vi "GroupUI.vi"() -> ()   [LabVIEW 2013, in "device.lvclass"]
uses:
  device.lvclass
  <vilib>/NI/Configuration Framework/Node/NodeRef.ctl
  <vilib>/NI/Configuration Framework/Node/NISE_CEF_Node.lvclass
  <vilib>/NI/AMC/Message Queue.ctl
  <vilib>/NI/AMC/Message.ctl
  <vilib>/NI/Tools/Keyed Array/KeyedArray.ctl
  <vilib>/NI/Configuration Framework/Node/UserEventRef.ctl
  <vilib>/NI/Configuration Framework/Controls/EventCluster.ctl
  database file/signal configuration.ctl
  J1939 Library/Configuration/TypeDefs/J1939 db frame direction.ctl
  device.lvclass/device.ctl
  device registry command.ctl
  <vilib>/NI/AMC/Create Single Message.vi
  <vilib>/NI/AMC/Update Message Routing Info.vi
  database file/J1939FullDB.vi
  <vilib>/NI/AMC/Send Message.vi
  <vilib>/NI/AMC/AMC.lvlib
  database file/database file.lvclass
  <vilib>/NI/Tools/Keyed Array/Tools_KeyedArray.lvlib
  <vilib>/NI/Configuration Framework/NISE_CEF_TreeControl.lvlib
  J1939 Library/J1939.lvlib
panel:
  in  "Direction":T1
  in  "Priority":u8
  in  "Transmit Time":dbl
  in  "Output Timing Type":u32(ring) items=["Cyclic Data", "Event Data"]
  out "information":string
  in  "Signals":T2[](array[typedef])
  in  "remove":bool
  in  "add":bool
  in  "Configured Frames (PGN)":i32(listbox)
  in  "Available Frames (PGN)":i32(listbox)
  in  "Source Address":u8
  in  "user event":T3
  in  "main queue":T4
  in  "node ref":T5
  # "Frame Settings"
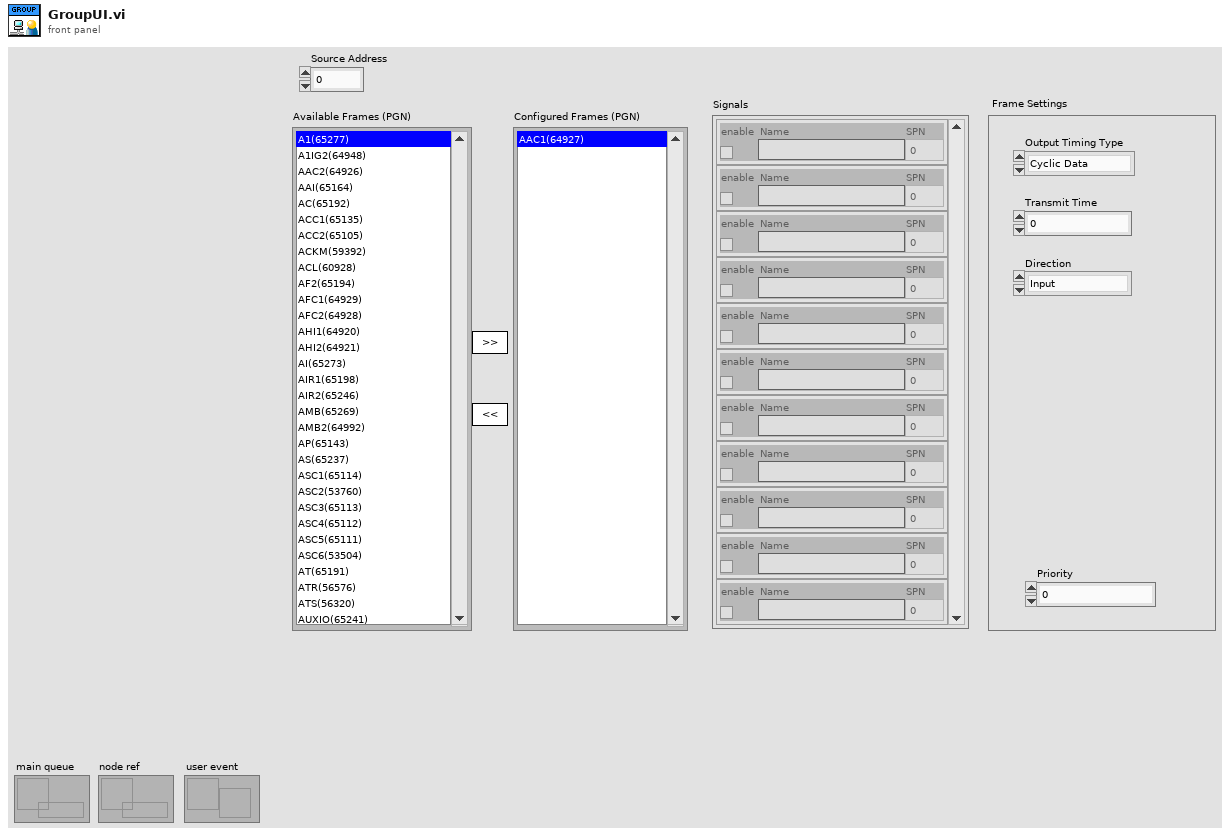
[diagram p1: front panel]
types:
  T1 = typedef "J1939.lvlib/J1939 db frame direction.ctl" = enum16{"Input", "Output", "Input+Output"}
  T2 = typedef "device.lvclass/signal configuration.ctl" = cluster{"enable":bool, "Name":string, "SPN":u32}
  T3 = typedef "NISE_CEF_Node.lvclass/UserEventRef.ctl" = refnum<user-event>
  T4 = typedef "AMC.lvlib/Message Queue.ctl" = refnum<queue>
  T5 = typedef "NISE_CEF_Node.lvclass/NodeRef.ctl" = refnum<data-value>
  T6 = typedef "J1939.lvlib/J1939 db.ctl" = cluster{"BaudRate":u32, "CAN.IoMode":u32, "J1939 Network Address":u8, "Name":u64, "frames":T7[]}
  T7 = typedef "J1939.lvlib/J1939 db frame.ctl" = cluster{"name":string, "Priority":u8, "PGN":u32, "Reserved Bit":u8, "Data page":u8, "PDU Format":u8, "PDU Specific":u8, "Source Address":u8, "PayldLen":u32, "signals":T8[], "Comment":string, "can timing type":u32, "transmit time":dbl, "direction":u16}
  T8 = typedef "J1939.lvlib/J1939 db signal.ctl" = cluster{"NameShort":string, "SPN":i32, "StartBit":u32, "NumBits":u32, "DataType":u32, "ByteOrdr":u32, "ScaleFac":dbl, "ScaleOff":dbl, "Max":dbl, "Min":dbl, "Default":dbl, "Unit":string, "Comment":string}
  T9 = typedef "device.lvclass/device registry command.ctl" = enum16{"add device", "remove device", "get next available"}
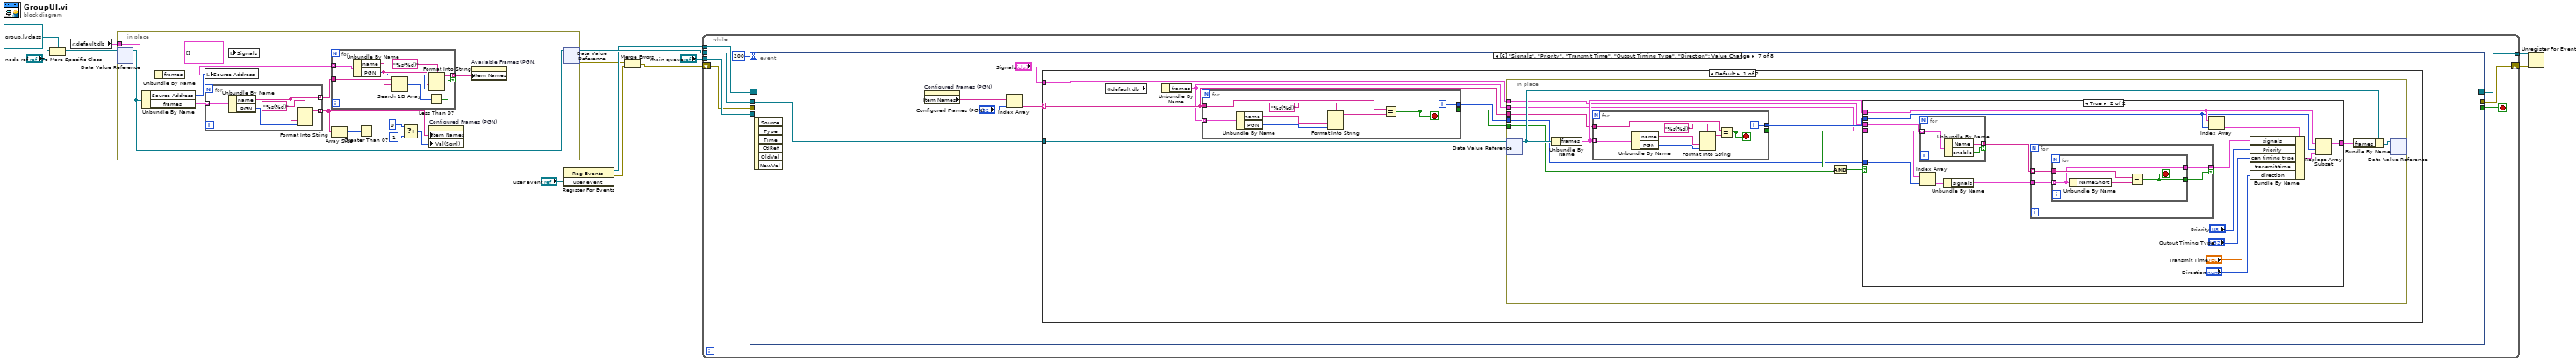
[diagram p0: block diagram]
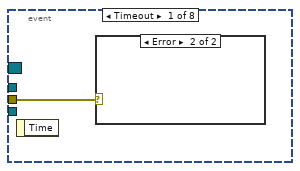
[diagram p2: hidden frame]
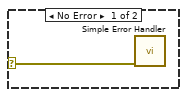
[diagram p3: hidden frame]
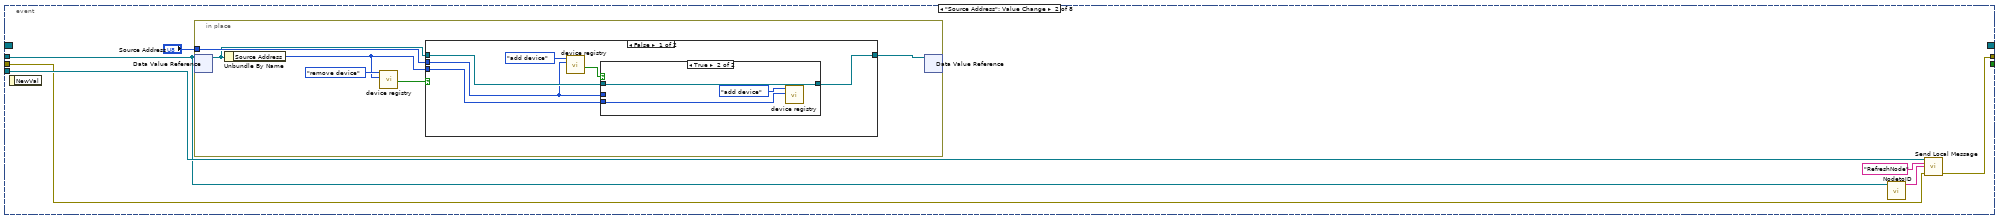
[diagram p4: hidden frame]
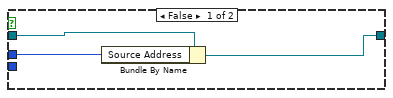
[diagram p5: hidden frame]
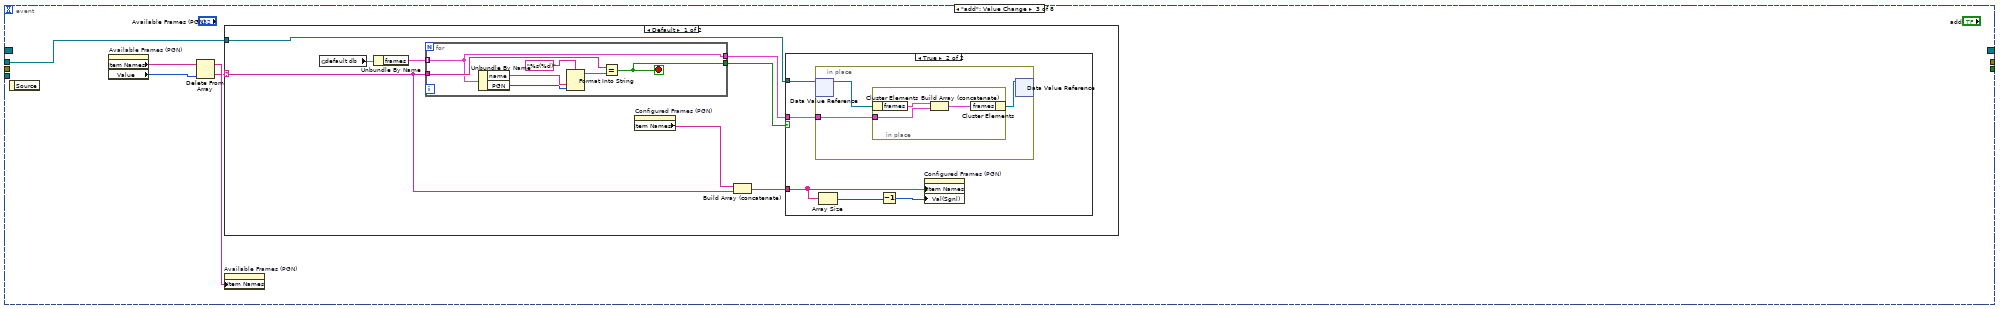
[diagram p7: hidden frame]
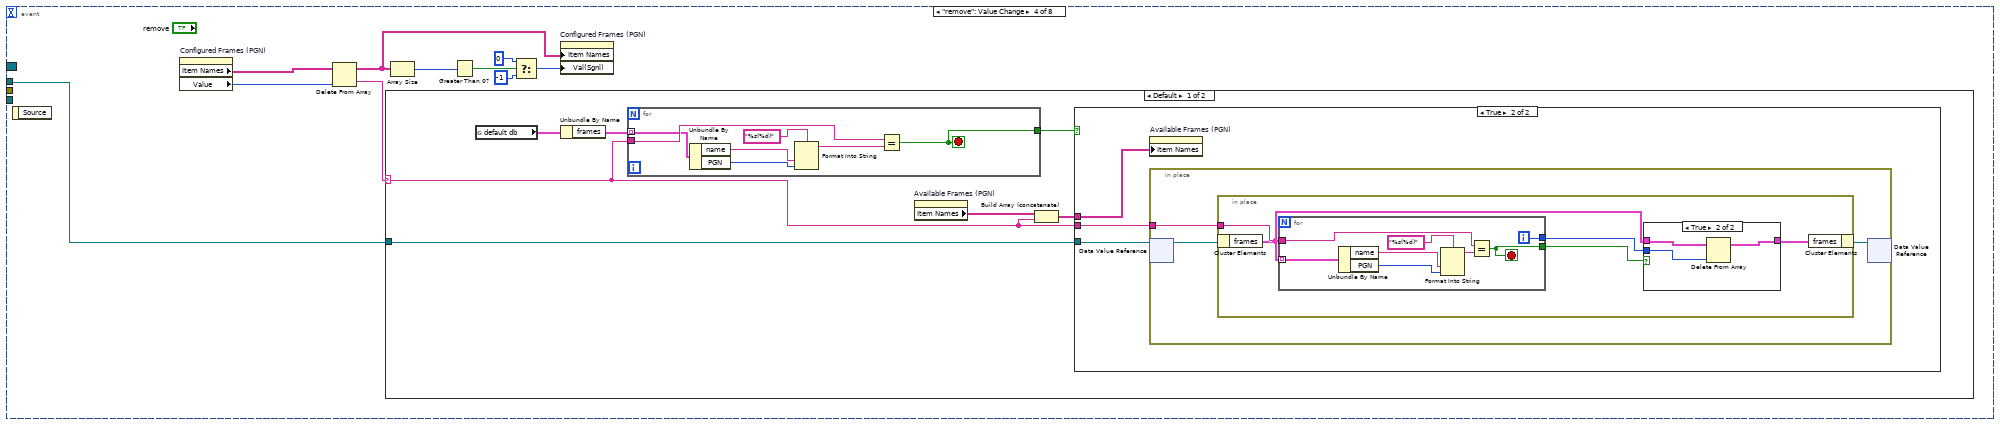
[diagram p10: hidden frame]
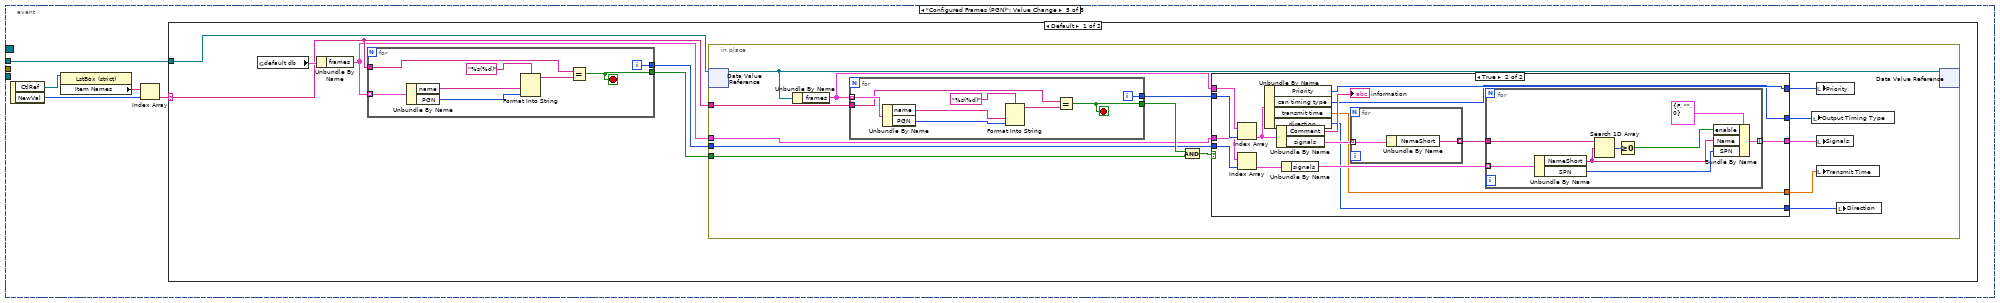
[diagram p14: hidden frame]
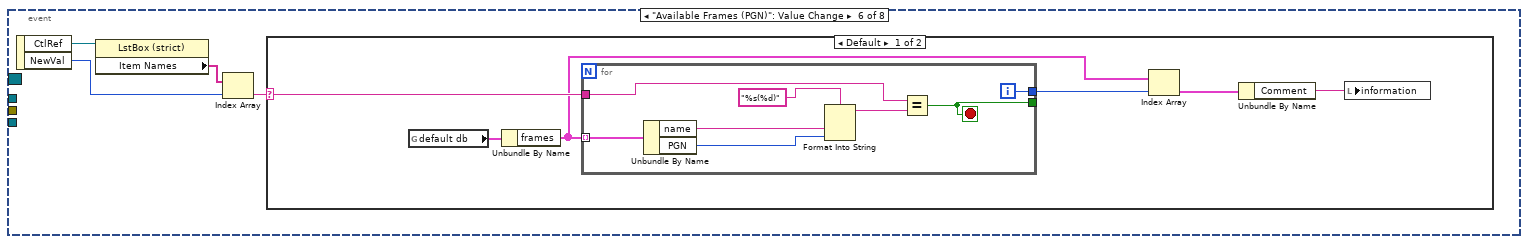
[diagram p17: hidden frame]
diagram:
  n1 = To More Specific Class(target class=refnum<data-value> refnum ("data value reference"), reference="node ref") -> (specific class reference=w6:refnum<data-value>)  [unwired: 1 in, 1 out]
  n2 = global read "J1939FullDB.vi" "default db"() -> (w1:T6)
  n3 = in-place {
    in-place-border: w1 -> [w18]
    n4 = in-place-dvr #1(w6) -> (w27:refnum<class "device.lvclass">)  [unwired: 1 out]
    n5 = Unbundle By Name(w27) -> ("Source Address"=w26:u8, "frames"=w25:T7[])
    n6 = Unbundle By Name(w18) -> ("frames"=w17:T7[])
    n7 = local write "Source Address"(w26) -> ()
    n8 = for {
      tunnel: w25 -> [w40] mode=indexing
      tunnel: [w37] -> w24 mode=indexing
      tunnel: [w36] -> w16 mode=indexing
      n9 = Unbundle By Name(w40) -> ("name"=w36:string, "PGN"=w39:u32)
      n10 = Format Into String(format string="%s(%d)", w36, w39) -> (resulting string=w37:string)  [unwired: 2 in, 1 out]
    }
    n11 = local write "Signals"(T2[] [] ("Signals")) -> ()
    n12 = for {
      tunnel: w17 -> [w35] mode=indexing
      tunnel: w16 -> [w34]
      tunnel: [w30] -> w15 mode=indexing if=w28
      n13 = Unbundle By Name(w35) -> ("name"=w32:string, "PGN"=w31:u32)
      n14 = Search 1D Array(1D array=w34, element=w32) -> (index of element=w29:i32)  [unwired: 1 in]
      n15 = Less Than 0?(x=w29) -> (x < 0?=w28:bool)
      n16 = Format Into String(format string="%s(%d)", w32, w31) -> (resulting string=w30:string)  [unwired: 2 in, 1 out]
    }
    n17 = Array Size(array=w24) -> (size(s)=w23:i32)
    n18 = Greater Than 0?(x=w23) -> (x > 0?=w22:bool)
    n19 = Select(t=0 ("Value (Signaling)"), s=w22, f=-1 ("Value (Signaling)")) -> (s? t:f=w20:i32)
    n20 = property on="Configured Frames (PGN)" class="LstBox (strict)"("Item Names"=w24, "Val(Sgnl)"=w20) -> ()  [unwired: 2 in, 2 out]
    n21 = property on="Available Frames (PGN)" class="LstBox (strict)"("Item Names"=w15) -> ()  [unwired: 2 in, 2 out]
    n22 = in-place-dvr #1(w27) -> (w13:refnum<data-value>, w3:errorcluster)
  }
  n23 = register-events("user event") -> (reference out=w10:refnum<event-registration>, error out=w4:errorcluster)  [unwired: 2 in]
  n24 = Merge Errors(w3, w4) -> (w2:errorcluster)
  n25 = while {
    tunnel: w13 -> [w48]
    tunnel: "main queue" -> [w47]
    tunnel: w10 -> [w45]
    tunnel: [w44] -> w9
    shift-right: [w42] -> w8
    shift-left: w2 -> [w41]
    stop <- w43 stop-if-true
    n26 = event shown="[6] \"Signals\", \"Priority\", \"Transmit Time\", \"Output Timing Type\", \"Direction\": Value Change" {
      selector: w45 -> [_ _ _ _ _ _ _ _]
      dyn-events: [_ _ _ _ _ _ _ _] -> w44
      timeout: 200 -> [_ _ _ _ _ _ _ _]
      tunnel: w48 -> [_ w55 w77 w114 w155 _ w239 _]
      tunnel: w47 -> [_ w56 _ _ _ _ _ _]
      tunnel: [_ _ _ _ _ _ _ TRUE] -> w43
      tunnel: [_ w53 _ _ _ _ _ _] -> w42
      tunnel: w41 -> [w49 w52 _ _ _ _ _ _]
      event Timeout {
        n27 = event-data() -> ()  [unwired: 1 in, 1 out]
        n28 = case shown="Error" w49 {
          selector: w49 -> [w50 _]
          frame No Error {
            n29 = call <vilib>:"Simple Error Handler.vi"("error in (no error)"=w50) -> ()  [unwired: 4 in, 5 out]
          }
          frame Error {
          }
        }
      }
      event "Source Address": Value Change {
        n30 = event-data() -> ()  [unwired: 1 in, 1 out]
        n31 = in-place {
          in-place-border: "Source Address" -> [w62]
          n32 = in-place-dvr #2(w55) -> (w61:refnum<class "device.lvclass">)  [unwired: 1 out]
          n33 = Unbundle By Name(w61) -> ("Source Address"=w58:u8)
          n34 = call "device registry.vi"("device"=w58, "command"=device_registry_command."remove device") -> ("Error?"=w59:bool)  [unwired: 8 in, 1 out]
          n35 = case shown="False" w59 {
            tunnel: [w69 w76] -> w63
            tunnel: w62 -> [w65 _]
            tunnel: w61 -> [w68 w76]
            tunnel: w58 -> [w64 _]
            frame False {
              n36 = call "device registry.vi"("device"=w65, "command"=device_registry_command."add device") -> ("Error?"=w66:bool)  [unwired: 8 in, 1 out]
              n37 = case shown="True" w66 {
                tunnel: [w72 w75] -> w69
                tunnel: w68 -> [w71 w75]
                tunnel: w65 -> [w70 _]
                tunnel: w64 -> [_ w73]
                frame False {
                  n38 = Bundle By Name(cluster=w71, "Source Address"=w70) -> (w72:refnum<class "device.lvclass">)
                }
                frame True {
                  n39 = call "device registry.vi"("device"=w73, "command"=device_registry_command."add device") -> ()  [unwired: 8 in, 2 out]
                }
              }
            }
            frame True {
            }
          }
          n40 = in-place-dvr #2(w63) -> ()  [unwired: 2 out]
        }
        n41 = call <vilib>:"NodetoID.vi"("node ref"=w55) -> ("ID"=w54:string)  [unwired: 9 in, 1 out]
        n42 = call <vilib>:"Send Local Message.vi"("message queue in"=w56, "message name"="RefreshNode" ("Message Name"), "message value"=w54, "error in"=w52) -> ("error out"=w53:errorcluster)  [unwired: 9 in, 2 out]
      }
      event "add": Value Change {
        n43 = event-data() -> ()  [unwired: 1 in, 1 out]
        n44 = property on="Available Frames (PGN)" class="LstBox (strict)"() -> ("Item Names"=w81:string[], "Value"=w80:i32)  [unwired: 2 in, 2 out]
        n45 = Delete From Array(array=w81, index=w80) -> (deleted portion=w78:string, array with subset deleted=w79:string[])  [unwired: 1 in]
        n46 = case shown="Default" w78 {
          selector: w78 -> [w86 _]
          tunnel: w77 -> [w83 _]
          frame Default {
            n47 = global read "J1939FullDB.vi" "default db"() -> (w88:T6)
            n48 = Unbundle By Name(w88) -> ("frames"=w87:T7[])
            n49 = for {
              tunnel: w87 -> [w101] mode=indexing
              tunnel: w86 -> [w103]
              tunnel: [w102] -> w85
              tunnel: [w101] -> w82
              stop <- w102 stop-if-true
              n50 = Unbundle By Name(w101) -> ("name"=w106:string, "PGN"=w105:u32)
              n51 = Format Into String(format string="%s(%d)", w106, w105) -> (resulting string=w104:string)  [unwired: 2 in, 1 out]
              n52 = Equal?(x=w103, y=w104) -> (x = y?=w102:bool)
            }
            n53 = property on="Configured Frames (PGN)" class="LstBox (strict)"() -> ("Item Names"=w89:string[])  [unwired: 2 in, 2 out]
            n54 = Build Array (concatenate)(w89, w86) -> (w84:string[])
            n55 = case shown="True" w85 {
              tunnel: w84 -> [_ w92]
              tunnel: w83 -> [_ w94]
              tunnel: w82 -> [_ w93]
              frame False {
              }
              frame True {
                n56 = in-place {
                  in-place-border: w93 -> [w95]
                  n57 = in-place-dvr #3(w94) -> (w97:refnum<class "device.lvclass">)  [unwired: 1 out]
                  n58 = in-place {
                    in-place-border: w95 -> [w99]
                    n59 = in-place-cluster #4(w97) -> ("frames"=w100:T7[])
                    n60 = Build Array (concatenate)(w100, w99) -> (w98:T7[])
                    n61 = in-place-cluster #4("frames"=w98) -> (w96:refnum<class "device.lvclass">)
                  }
                  n62 = in-place-dvr #3(w96) -> ()  [unwired: 2 out]
                }
                n63 = Array Size(array=w92) -> (size(s)=w91:i32)
                n64 = Decrement(x=w91) -> (x-1=w90:i32)
                n65 = property on="Configured Frames (PGN)" class="LstBox (strict)"("Item Names"=w92, "Val(Sgnl)"=w90) -> ()  [unwired: 2 in, 2 out]
              }
            }
          }
          frame "" {
          }
        }
        n66 = property on="Available Frames (PGN)" class="LstBox (strict)"("Item Names"=w79) -> ()  [unwired: 2 in, 2 out]
      }
      event "remove": Value Change {
        n67 = event-data() -> ()  [unwired: 1 in, 1 out]
        n68 = property on="Configured Frames (PGN)" class="LstBox (strict)"() -> ("Item Names"=w117:string[], "Value"=w116:i32)  [unwired: 2 in, 2 out]
        n69 = Delete From Array(array=w117, index=w116) -> (deleted portion=w115:string, array with subset deleted=w109:string[])  [unwired: 1 in]
        n70 = case shown="Default" w115 {
          selector: w115 -> [w118 _]
          tunnel: w114 -> [w119 _]
          frame Default {
            n71 = global read "J1939FullDB.vi" "default db"() -> (w123:T6)
            n72 = Unbundle By Name(w123) -> ("frames"=w122:T7[])
            n73 = for {
              tunnel: w122 -> [w148] mode=indexing
              tunnel: w118 -> [w150]
              tunnel: [w149] -> w121
              stop <- w149 stop-if-true
              n74 = Unbundle By Name(w148) -> ("name"=w153:string, "PGN"=w152:u32)
              n75 = Format Into String(format string="%s(%d)", w153, w152) -> (resulting string=w151:string)  [unwired: 2 in, 1 out]
              n76 = Equal?(x=w150, y=w151) -> (x = y?=w149:bool)
            }
            n77 = property on="Available Frames (PGN)" class="LstBox (strict)"() -> ("Item Names"=w124:string[])  [unwired: 2 in, 2 out]
            n78 = Build Array (concatenate)(w124, w118) -> (w120:string[])
            n79 = case shown="True" w121 {
              tunnel: w120 -> [_ w127]
              tunnel: w119 -> [_ w126]
              tunnel: w118 -> [_ w125]
              frame False {
              }
              frame True {
                n80 = property on="Available Frames (PGN)" class="LstBox (strict)"("Item Names"=w127) -> ()  [unwired: 2 in, 2 out]
                n81 = in-place {
                  in-place-border: w125 -> [w128]
                  n82 = in-place-dvr #5(w126) -> (w130:refnum<class "device.lvclass">)  [unwired: 1 out]
                  n83 = in-place {
                    in-place-border: w128 -> [w135]
                    n84 = in-place-cluster #6(w130) -> ("frames"=w132:T7[])
                    n85 = for {
                      tunnel: w132 -> [w141] mode=indexing
                      tunnel: w135 -> [w143]
                      tunnel: [w142] -> w134
                      tunnel: [w140] -> w131
                      i -> [w140]
                      stop <- w142 stop-if-true
                      n86 = Unbundle By Name(w141) -> ("name"=w146:string, "PGN"=w145:u32)
                      n87 = Format Into String(format string="%s(%d)", w146, w145) -> (resulting string=w144:string)  [unwired: 2 in, 1 out]
                      n88 = Equal?(x=w143, y=w144) -> (x = y?=w142:bool)
                    }
                    n89 = case shown="True" w134 {
                      tunnel: [w136 w137] -> w133
                      tunnel: w132 -> [w136 w139]
                      tunnel: w131 -> [_ w138]
                      frame False {
                      }
                      frame True {
                        n90 = Delete From Array(array=w139, index=w138) -> (array with subset deleted=w137:T7[])  [unwired: 1 in, 1 out]
                      }
                    }
                    n91 = in-place-cluster #6("frames"=w133) -> (w129:refnum<class "device.lvclass">)
                  }
                  n92 = in-place-dvr #5(w129) -> ()  [unwired: 2 out]
                }
              }
            }
          }
          frame "" {
          }
        }
        n93 = Array Size(array=w109) -> (size(s)=w110:i32)
        n94 = Greater Than 0?(x=w110) -> (x > 0?=w111:bool)
        n95 = Select(t=0 ("Value (Signaling)"), s=w111, f=-1 ("Value (Signaling)")) -> (s? t:f=w108:i32)
        n96 = property on="Configured Frames (PGN)" class="LstBox (strict)"("Item Names"=w109, "Val(Sgnl)"=w108) -> ()  [unwired: 2 in, 2 out]
      }
      event "Configured Frames (PGN)": Value Change {
        n97 = event-data() -> ("CtlRef"=w159:refnum<vi>, "NewVal"=w156:i32)  [unwired: 1 in]
        n98 = property class="LstBox (strict)"(reference=w159) -> ("Item Names"=w158:string[])  [unwired: 1 in, 2 out]
        n99 = Index Array(array=w158, index=w156) -> (element=w157:string)
        n100 = case shown="Default" w157 {
          selector: w157 -> [w164 _]
          tunnel: w155 -> [w160 _]
          frame Default {
            n101 = global read "J1939FullDB.vi" "default db"() -> (w165:T6)
            n102 = Unbundle By Name(w165) -> ("frames"=w161:T7[])
            n103 = for {
              tunnel: w161 -> [w167] mode=indexing
              tunnel: w164 -> [w169]
              tunnel: [w168] -> w163
              tunnel: [w166] -> w162
              i -> [w166]
              stop <- w168 stop-if-true
              n104 = Unbundle By Name(w167) -> ("name"=w172:string, "PGN"=w171:u32)
              n105 = Format Into String(format string="%s(%d)", w172, w171) -> (resulting string=w170:string)  [unwired: 2 in, 1 out]
              n106 = Equal?(x=w169, y=w170) -> (x = y?=w168:bool)
            }
            n107 = in-place {
              in-place-border: w164 -> [w183]
              in-place-border: w163 -> [w181]
              in-place-border: w162 -> [w180]
              in-place-border: w161 -> [w179]
              n108 = in-place-dvr #7(w160) -> (w184:refnum<class "device.lvclass">)  [unwired: 1 out]
              n109 = Unbundle By Name(w184) -> ("frames"=w186:T7[])
              n110 = for {
                tunnel: w186 -> [w215] mode=indexing
                tunnel: [w216] -> w187
                tunnel: [w214] -> w185
                tunnel: w183 -> [w213]
                i -> [w214]
                stop <- w216 stop-if-true
                n111 = Unbundle By Name(w215) -> ("name"=w219:string, "PGN"=w218:u32)
                n112 = Format Into String(format string="%s(%d)", w219, w218) -> (resulting string=w217:string)  [unwired: 2 in, 1 out]
                n113 = Equal?(x=w213, y=w217) -> (x = y?=w216:bool)
              }
              n114 = And(x=w187, y=w181) -> (x .and. y?=w182:bool)
              n115 = case shown="True" w182 {
                tunnel: w186 -> [_ w202]
                tunnel: w185 -> [_ w201]
                tunnel: w180 -> [_ w199]
                tunnel: w179 -> [_ w200]
                tunnel: [_ w194] -> w178
                tunnel: [_ w191] -> w177
                tunnel: [_ w190] -> w176
                tunnel: [_ w189] -> w175
                tunnel: [_ w188] -> w174
                frame False {
                }
                frame True {
                  n116 = Index Array(array=w202, index=w201) -> (element=w192:T7)
                  n117 = Index Array(array=w200, index=w199) -> (element=w198:T7)
                  n118 = Unbundle By Name(w192) -> ("Priority"=w191:u8, "can timing type"=w190:u32, "transmit time"=w189:dbl, "direction"=w188:u16)
                  n119 = Unbundle By Name(w192) -> ("Comment"=→"information":string, "signals"=w196:T8[])
                  n120 = Unbundle By Name(w198) -> ("signals"=w197:T8[])
                  n121 = for {
                    tunnel: w196 -> [w204] mode=indexing
                    tunnel: [w203] -> w195 mode=indexing
                    n122 = Unbundle By Name(w204) -> ("NameShort"=w203:string)
                  }
                  n123 = for {
                    tunnel: w197 -> [w211] mode=indexing
                    tunnel: w195 -> [w209]
                    tunnel: [w205] -> w194 mode=indexing
                    n124 = Unbundle By Name(w211) -> ("NameShort"=w208:string, "SPN"=w210:i32)
                    n125 = Search 1D Array(1D array=w209, element=w208) -> (index of element=w207:i32)  [unwired: 1 in]
                    n126 = Greater Or Equal To 0?(x=w207) -> (x >= 0?=w206:bool)
                    n127 = Bundle By Name(cluster=T2 {"enable"=FALSE, "Name"="", "SPN"=0} ("signal"), "enable"=w206, "Name"=w208, "SPN"=w210) -> (w205:T2)
                  }
                }
              }
              n128 = local write "Output Timing Type"(w176) -> ()
              n129 = local write "Priority"(w177) -> ()
              n130 = local write "Signals"(w178) -> ()
              n131 = local write "Transmit Time"(w175) -> ()
              n132 = local write "Direction"(w174) -> ()
              n133 = in-place-dvr #7(w184) -> ()  [unwired: 2 out]
            }
          }
          frame "" {
          }
        }
      }
      event "Available Frames (PGN)": Value Change {
        n134 = event-data() -> ("CtlRef"=w224:refnum<vi>, "NewVal"=w221:i32)  [unwired: 1 in]
        n135 = property class="LstBox (strict)"(reference=w224) -> ("Item Names"=w223:string[])  [unwired: 1 in, 2 out]
        n136 = Index Array(array=w223, index=w221) -> (element=w222:string)
        n137 = case shown="Default" w222 {
          selector: w222 -> [w229 _]
          frame Default {
            n138 = global read "J1939FullDB.vi" "default db"() -> (w230:T6)
            n139 = Unbundle By Name(w230) -> ("frames"=w227:T7[])
            n140 = for {
              tunnel: w227 -> [w232] mode=indexing
              tunnel: w229 -> [w234]
              tunnel: [w233] -> _
              tunnel: [w231] -> w226
              i -> [w231]
              stop <- w233 stop-if-true
              n141 = Unbundle By Name(w232) -> ("name"=w237:string, "PGN"=w236:u32)
              n142 = Format Into String(format string="%s(%d)", w237, w236) -> (resulting string=w235:string)  [unwired: 2 in, 1 out]
              n143 = Equal?(x=w234, y=w235) -> (x = y?=w233:bool)
            }
            n144 = Index Array(array=w227, index=w226) -> (element=w228:T7)
            n145 = Unbundle By Name(w228) -> ("Comment"=w225:string)
            n146 = local write "information"(w225) -> ()
          }
          frame "" {
          }
        }
      }
      event "Signals", "Priority", "Transmit Time", "Output Timing Type": Value Change {
        n147 = event-data() -> ()  [unwired: 1 in, 6 out]
        n148 = property on="Configured Frames (PGN)" class="LstBox (strict)"() -> ("Item Names"=w242:string[])  [unwired: 2 in, 2 out]
        n149 = Index Array(array=w242, index="Configured Frames (PGN)") -> (element=w243:string)
        n150 = case shown="Default" w243 {
          selector: w243 -> [w249 _]
          tunnel: "Signals" -> [w245 _]
          tunnel: w239 -> [w244 _]
          frame Default {
            n151 = global read "J1939FullDB.vi" "default db"() -> (w250:T6)
            n152 = Unbundle By Name(w250) -> ("frames"=w246:T7[])
            n153 = for {
              tunnel: w246 -> [w252] mode=indexing
              tunnel: w249 -> [w254]
              tunnel: [w253] -> w248
              tunnel: [w251] -> w247
              i -> [w251]
              stop <- w253 stop-if-true
              n154 = Unbundle By Name(w252) -> ("name"=w257:string, "PGN"=w256:u32)
              n155 = Format Into String(format string="%s(%d)", w257, w256) -> (resulting string=w255:string)  [unwired: 2 in, 1 out]
              n156 = Equal?(x=w254, y=w255) -> (x = y?=w253:bool)
            }
            n157 = in-place {
              in-place-border: w249 -> [w266]
              in-place-border: w248 -> [w264]
              in-place-border: w247 -> [w263]
              in-place-border: w246 -> [w262]
              in-place-border: w245 -> [w259]
              n158 = in-place-dvr #8(w244) -> (w267:refnum<class "device.lvclass">)  [unwired: 1 out]
              n159 = Unbundle By Name(w267) -> ("frames"=w269:T7[])
              n160 = for {
                tunnel: w269 -> [w301] mode=indexing
                tunnel: [w302] -> w270
                tunnel: [w300] -> w268
                tunnel: w266 -> [w299]
                i -> [w300]
                stop <- w302 stop-if-true
                n161 = Unbundle By Name(w301) -> ("name"=w305:string, "PGN"=w304:u32)
                n162 = Format Into String(format string="%s(%d)", w305, w304) -> (resulting string=w303:string)  [unwired: 2 in, 1 out]
                n163 = Equal?(x=w299, y=w303) -> (x = y?=w302:bool)
              }
              n164 = And(x=w270, y=w264) -> (x .and. y?=w265:bool)
              n165 = case shown="True" w265 {
                tunnel: w269 -> [w271 w284]
                tunnel: w268 -> [_ w283]
                tunnel: w263 -> [_ w286]
                tunnel: w262 -> [_ w287]
                tunnel: [w271 w282] -> w260
                tunnel: w259 -> [_ w281]
                frame False {
                }
                frame True {
                  n166 = for {
                    tunnel: w281 -> [w298] mode=indexing
                    tunnel: [w297] -> w277 mode=indexing if=w296
                    n167 = Unbundle By Name(w298) -> ("Name"=w297:string, "enable"=w296:bool)
                  }
                  n168 = Index Array(array=w287, index=w286) -> (element=w285:T7)
                  n169 = Unbundle By Name(w285) -> ("signals"=w278:T8[])
                  n170 = for {
                    tunnel: w278 -> [w291]
                    tunnel: w277 -> [w290] mode=indexing
                    tunnel: [w289] -> w276 mode=indexing if=w288
                    n171 = for {
                      tunnel: w291 -> [w293] mode=indexing
                      tunnel: w290 -> [w294]
                      tunnel: [w293] -> w289
                      tunnel: [w292] -> w288
                      stop <- w292 stop-if-true
                      n172 = Unbundle By Name(w293) -> ("NameShort"=w295:string)
                      n173 = Equal?(x=w294, y=w295) -> (x = y?=w292:bool)
                    }
                  }
                  n174 = Index Array(array=w284, index=w283) -> (element=w280:T7)
                  n175 = Bundle By Name(cluster=w280, "signals"=w276, "Priority"="Priority", "can timing type"="Output Timing Type", "transmit time"="Transmit Time", "direction"="Direction") -> (w279:T7)
                  n176 = Replace Array Subset(array=w284, new element=w279, index=w283) -> (w282:T7[])
                }
              }
              n177 = Bundle By Name(cluster=w267, "frames"=w260) -> (w261:refnum<class "device.lvclass">)
              n178 = in-place-dvr #8(w261) -> ()  [unwired: 2 out]
            }
          }
          frame "" {
          }
        }
      }
      event User Event {
        n179 = event-data() -> ()  [unwired: 1 in, 1 out]
      }
    }
  }
  n180 = Unregister For Events(event registration refnum=w9, error in=w8) -> ()  [unwired: 1 out]
